vi "lfm_rate_calculate.vi"(8 "SPC":dbl, 9 "fs":dbl=200000000.0 format="%#_13p", 10 "pw":dbl=200.0 format="%#_13g", 11 "f span":dbl) -> (3 "integer (fxp cast)":u32)   [LabVIEW 2021]
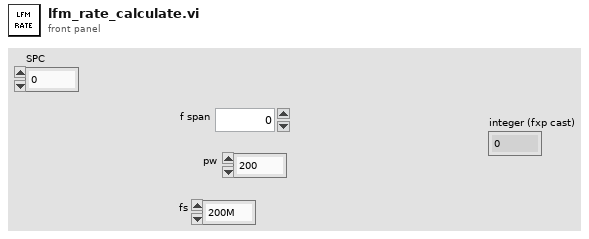
[diagram p1: front panel]
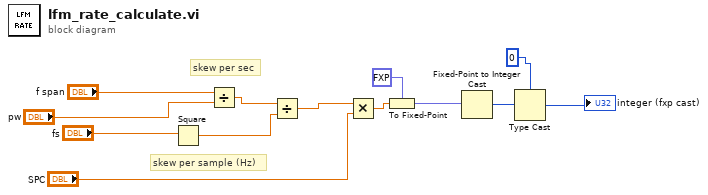
[diagram p0: block diagram]
diagram:
  # "skew per sample (Hz)"
  # "skew per sec"
  n1 = Square(x="fs") -> (x^2=w9:dbl)
  n2 = Divide(x="f span", y="pw") -> (x/y=w13:dbl)
  n3 = Divide(x=w13, y=w9) -> (x/y=w6:dbl)
  n4 = Multiply(x=w6, y="SPC") -> (x*y=w5:dbl)
  n5 = To Fixed-Point(fixed-point type=fxp<+/-,32,-16> 0.0, number=w5) -> (fixed-point=w8:fxp<+/-,32,-16>)
  n6 = Fixed-Point to Integer Cast(1:w8) -> (0:w3:i32)
  n7 = Type Cast(type=u32 0, x=w3) -> (*(type *) &x=→"integer (fxp cast)":u32)
